vi "Close Motor Communication_Vector.vi"(8 "error in (no error)":errorcluster, 11 "motor communication in":refnum<class "NI_Robotics_Motor Communication.lvclass">[](array[class])) -> (0 "error out":errorcluster)   [LabVIEW 2017, in "NI_Robotics_Motor Communication.lvclass"]
doc: "Terminates a communication session between a motor and the wheel the motor controls. Wire data to the <B>motor communication in</B> input to determine the polymorphic instance to use or manually select the instance."
uses:
  <vilib>/robotics/Actuation/Motor Communication/NI_Robotics_Motor Communication.lvclass
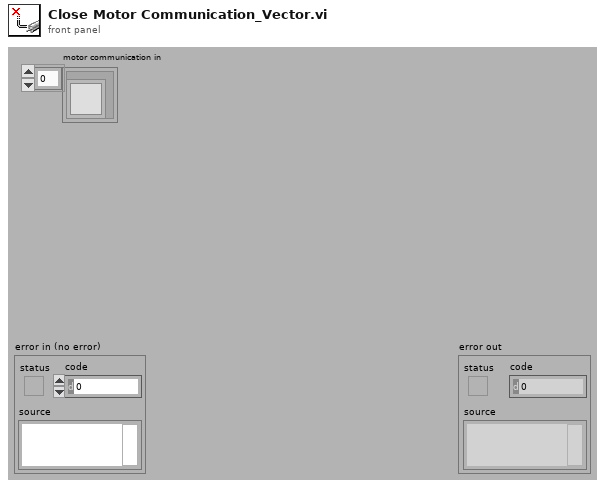
[diagram p1: front panel]
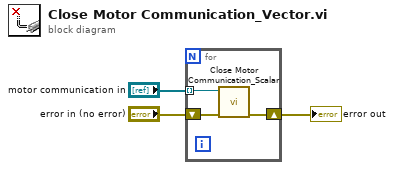
[diagram p0: block diagram]
diagram:
  n1 = for {
    tunnel: "motor communication in" -> [w6] mode=indexing
    shift-right: [w4] -> w1
    shift-left: "error in (no error)" -> [w5]
    n2 = call <vilib>:"Close Motor Communication_Scalar.vi"("error in (no error)"=w5, "motor communication in"=w6) -> ("error out"=w4:errorcluster)  [unwired: 9 in]
  }
  "error out" <- w1
